vi "Handle Last Ack Core.vi"(4 "error in":errorcluster, 6 "Last Ack":refnum<class "Last Ack.lvclass">, 7 "Study Actor in":refnum<class "Study Actor.lvclass">) -> (0 "error out":errorcluster, 3 "Study Actor out":refnum<class "Study Actor.lvclass">)   [LabVIEW 2023, in "Study Actor.lvlib" / "Study Actor.lvclass"]
doc: "(<B>Filename</B>: Actor Framework.lvlib:Actor.lvclass:Handle Last Ack Core.vi)\n\nDefines how the caller actor responds to the Last Ack message from a nested actor. The Last Ack message is the final message a nested actor sends to its caller before it shuts down. The message contains information about the final state of the nested actor.\n\nBy default, this method does nothing except return any error the nested actor sent. A descendant class may override this method to define behavior."
uses:
  Study Actor.lvclass
  <vilib>/ActorFramework/LastAck/Last Ack.lvclass
  Study Actor.lvclass/Study Actor.ctl
  <vilib>/ActorFramework/LastAck/Last Ack.lvclass/Last Ack.ctl
  <vilib>/MGI/Panel Manager/Panel Actor/Panel Actor/Panel Actor.lvclass
  <vilib>/ActorFramework/Actor/Actor.lvclass
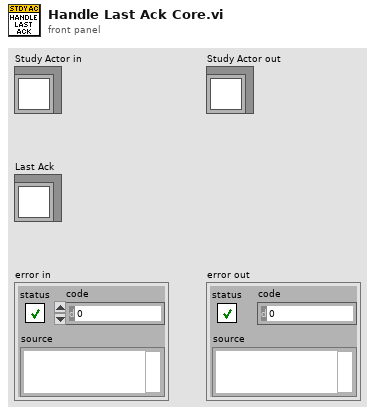
[diagram p1: front panel]
types:
  T1 = map{string, refnum<class "Message Enqueuer.lvclass">}
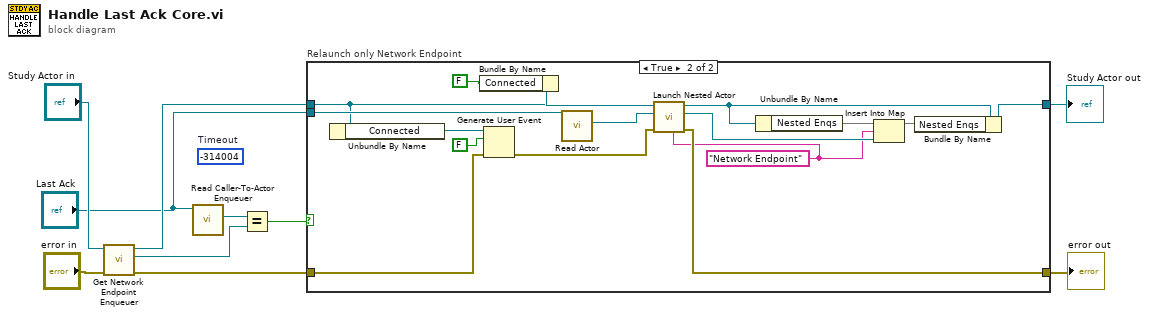
[diagram p0: block diagram]
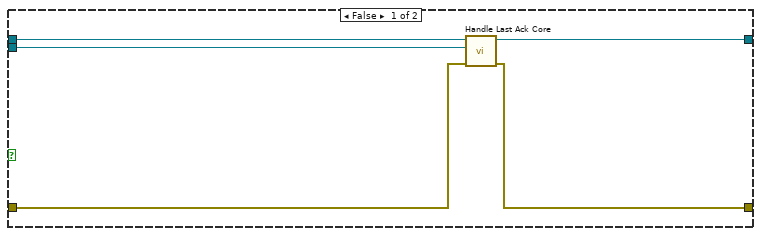
[diagram p2: hidden frame]
diagram:
  (unwired) -314004  # Timeout
  n1 = call "Get Network Endpoint Enqueuer.vi"("error in"="error in", "Study Actor in"="Study Actor in") -> ("error out"=w7:errorcluster, "Network Endpoint Enqueuer"=w2:refnum<class "Message Enqueuer.lvclass">, "Study Actor out"=w6:refnum<class "Study Actor.lvclass">)  [unwired: 6 in, 1 out]
  n2 = call <vilib>:"Read Caller-To-Actor Enqueuer.vi"("Last Ack"="Last Ack") -> ("Caller-to-Actor Enqueuer"=w3:refnum<class "Message Enqueuer.lvclass">)  [unwired: 10 in]
  n3 = Equal?(x=w3, y=w2) -> (x = y?=w1:bool)
  n4 = case "Relaunch only Network Endpoint" shown="True" w1 {
    tunnel: w6 -> [w15 w20]
    tunnel: [w13 w31] -> w8
    tunnel: [w14 w28] -> w9
    tunnel: "Last Ack" -> [w12 w25]
    tunnel: w7 -> [w11 w17]
    frame False {
      n5 = call-parent "Handle Last Ack Core.vi"("error in (no error)"=w11, "Last Ack"=w12, "Actor in"=w15) -> ("error out"=w13:errorcluster, "Actor out"=w14:refnum<class "Study Actor.lvclass">)  [unwired: 3 in]
    }
    frame True {
      w26 = "Network Endpoint" ("key")
      n6 = Unbundle By Name(w20) -> ("Connected"=w19:refnum<user-event>)
      n7 = Bundle By Name(cluster=w20, "Connected"=FALSE) -> (w22:refnum<class "Study Actor.lvclass">)
      n8 = Generate User Event(user event=w19, event data cluster=FALSE, error in=w17) -> (error out=w16:errorcluster)  [unwired: 1 in, 1 out]
      n9 = call <vilib>:"Read Actor.vi"("Last Ack"=w25) -> ("Actor"=w24:refnum<class "Actor.lvclass">)  [unwired: 10 in]
      n10 = call <vilib>:"Launch Nested Actor.vi"("Debug Alias"=w26, "error in (no error)"=w16, "Nested Actor"=w24, "Caller Actor in"=w22) -> ("error out"=w31:errorcluster, "Nested Actor's Enqueuer"=w29:refnum<class "Message Enqueuer.lvclass">, "Caller Actor out"=w30:refnum<class "Study Actor.lvclass">)  [unwired: 5 in]
      n11 = Unbundle By Name(w30) -> ("Nested Enqs"=w23:T1)
      n12 = Insert Into Map(map in=w23, key=w26, value=w29) -> (map out=w27:T1)  [unwired: 2 out]
      n13 = Bundle By Name(cluster=w30, "Nested Enqs"=w27) -> (w28:refnum<class "Study Actor.lvclass">)
    }
  }
  "Study Actor out" <- w9
  "error out" <- w8
